vi "TCPIPmain.vi"(5 "data":T1, 6 "config":T3, 7 "error in":errorcluster, 8 "data in":string, 9 "targer":enum16{"driver", "loader"}(ring), 10 "Enum":T4) -> (0 "error out":errorcluster, 1 "LED":bool[](array[boolean]), 2 "data out":T1, 3 "Data?":bool[](array[boolean]))   [LabVIEW 2015]
uses:
  TCPIP_enum.ctl
  TCPIPconfig.ctl
  Ctrls/data out array.ctl
  Ctrls/data out.ctl
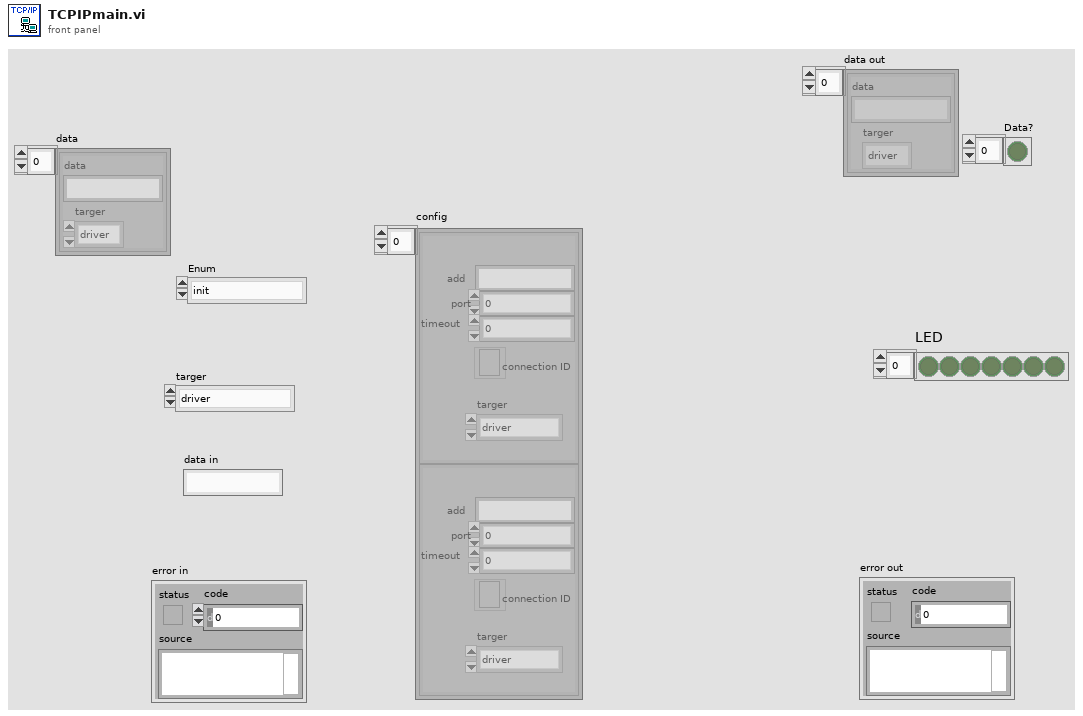
[diagram p1: front panel]
types:
  T1 = typedef "data out array.ctl" = T2[]
  T2 = typedef "data out.ctl" = cluster{"data":string, "targer":enum16{"driver", "loader"}}
  T3 = typedef "TCPIPconfig.ctl" = cluster{"add":string, "port":u32, "timeout":u16, "connection ID":refnum<k5>, "targer":enum16{"driver", "loader"}}[]
  T4 = typedef "TCPIP_enum.ctl" = enum16{"init", "connect", "command", "write", "read", "close", "null"}
  T5 = cluster{"data":string, "targer":enum16{"driver", "loader"}}
  T6 = cluster{"add":string, "port":u32, "timeout":u16, "connection ID":refnum<k5>, "targer":enum16{"driver", "loader"}}
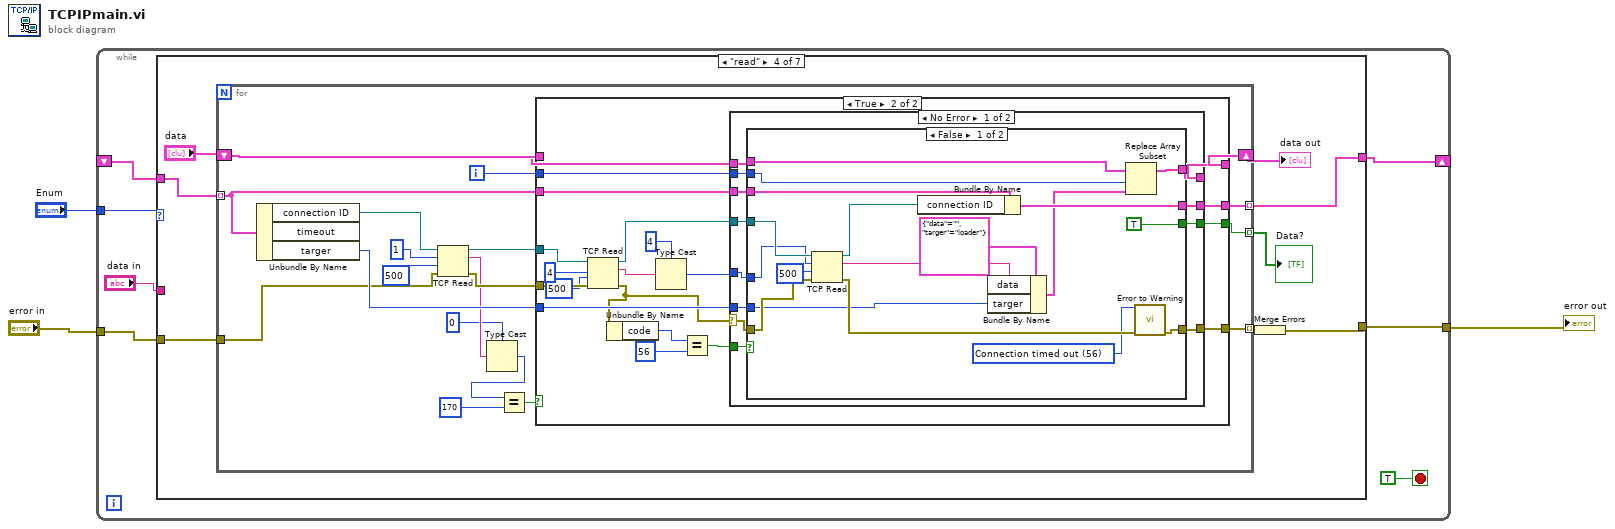
[diagram p0: block diagram]
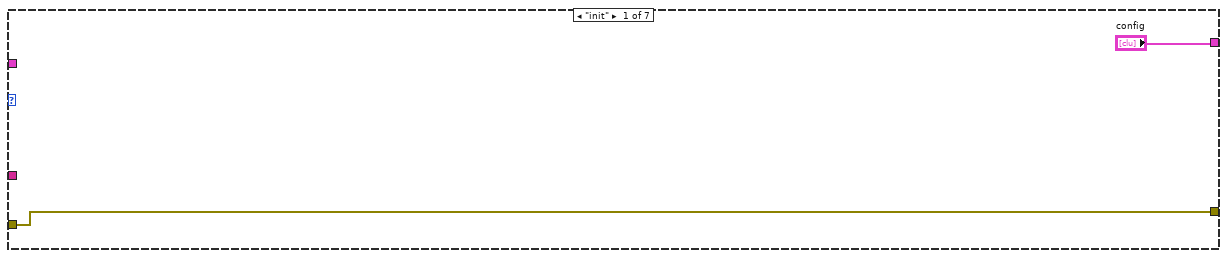
[diagram p2: hidden frame]
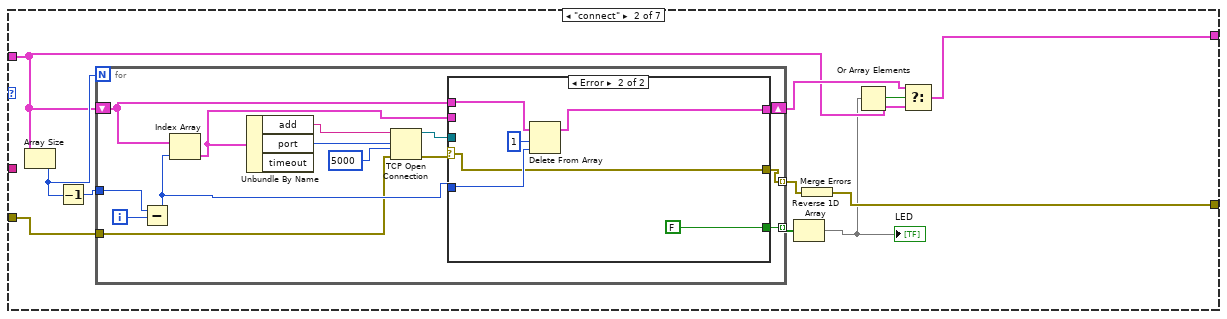
[diagram p3: hidden frame]
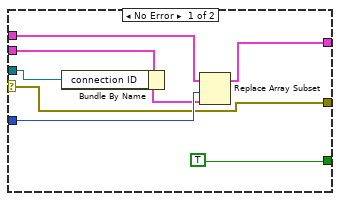
[diagram p4: hidden frame]
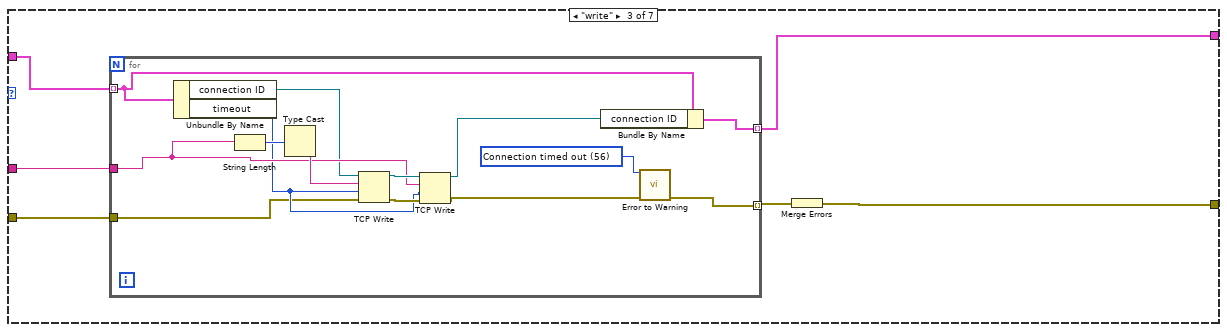
[diagram p5: hidden frame]
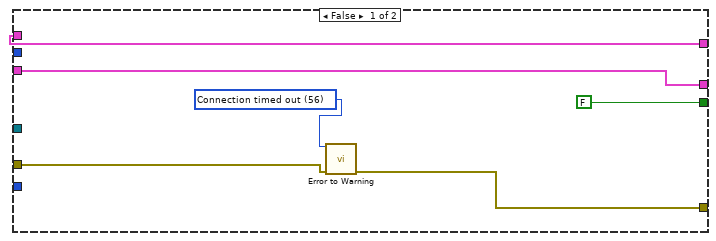
[diagram p6: hidden frame]
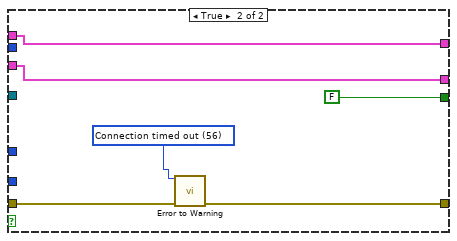
[diagram p7: hidden frame]
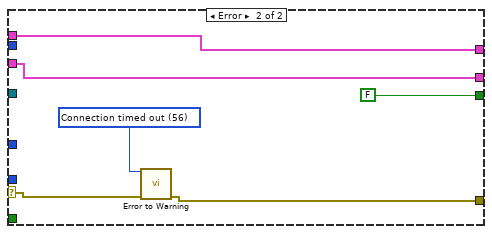
[diagram p8: hidden frame]
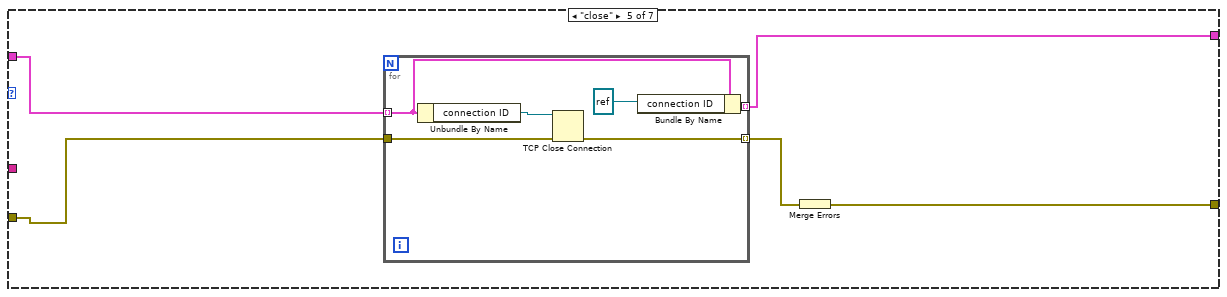
[diagram p9: hidden frame]
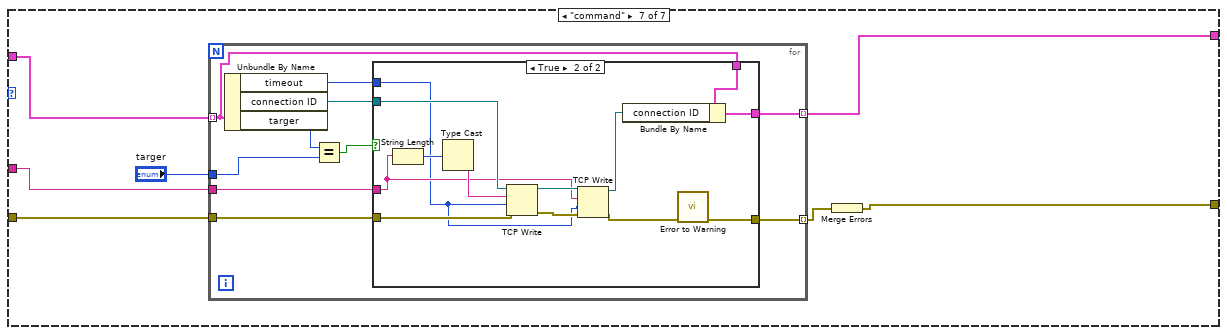
[diagram p11: hidden frame]
diagram:
  n1 = while {
    shift-right: [w8] -> _
    shift-left: _ -> [w7]
    tunnel: [w6] -> w2
    tunnel: "error in" -> [w5]
    tunnel: "Enum" -> [w9]
    stop <- TRUE stop-if-true
    n2 = case shown="\"read\"" w9 {
      tunnel: ["config" w14 w56 w78 w167 w179 w182] -> w8
      tunnel: w7 -> [_ w15 w57 w79 w171 w179 w186]
      tunnel: [w11 w20 w54 w76 w168 w178 w181] -> w6
      tunnel: w5 -> [w11 w22 w53 w75 w170 w178 w184]
      tunnel: "data in" -> [_ _ w52 _ _ _ w183]
      frame "init" {
      }
      frame "connect" {
        n3 = Array Size(array=w15) -> (size(s)=w19:i32)
        n4 = Decrement(x=w19) -> (x-1=w23:i32)
        n5 = for {
          N: w19 -> [_]
          shift-right: [w29] -> w16
          shift-left: w15 -> [w33]
          tunnel: w23 -> [w31]
          tunnel: w22 -> [w28]
          tunnel: [w27] -> w21 mode=indexing
          tunnel: [w26] -> w18 mode=indexing
          i -> [w32]
          n6 = Subtract(x=w31, y=w32) -> (x-y=w30:i32)
          n7 = Index Array(array=w33, index=w30) -> (element=w34:T6)
          n8 = Unbundle By Name(w34) -> ("add"=w37:string, "port"=w25:u32)  [unwired: 1 out]
          n9 = TCP Open Connection(address=w37, remote port or service name=w25, timeout ms (60000)=5000, error in (no error)=w28) -> (connection ID=w36:refnum<k5>, error out=w35:errorcluster)  [unwired: 1 in]
          n10 = case shown="Error" w35 {
            selector: w35 -> [w39 w47]
            tunnel: w36 -> [w45 _]
            tunnel: w34 -> [w44 _]
            tunnel: w33 -> [w43 w51]
            tunnel: w30 -> [w42 w49]
            tunnel: [w40 w48] -> w29
            tunnel: [w39 w47] -> w27
            tunnel: [TRUE FALSE] -> w26
            frame No Error {
              n11 = Bundle By Name(cluster=w44, "connection ID"=w45) -> (w41:T6)
              n12 = Replace Array Subset "Replace Array Subset"(array=w43, new element=w41, index=w42) -> (w40:T3)
            }
            frame Error {
              n13 = Delete From Array(array=w51, length=1, index=w49) -> (array with subset deleted=w48:T3)  [unwired: 1 out]
            }
          }
        }
        n14 = Reverse 1D Array(array=w18) -> (reversed array=w13:bool[])
        "LED" <- w13
        n15 = Merge Errors(w21) -> (w20:errorcluster)
        n16 = Or Array Elements(Boolean array=w13) -> (logical OR=w17:bool)
        n17 = Select(t=w16, s=w17, f=w15) -> (s? t:f=w14:T3)
      }
      frame "write" {
        n18 = for {
          tunnel: w57 -> [w63] mode=indexing
          tunnel: w52 -> [w66]
          tunnel: [w61] -> w56 mode=indexing
          tunnel: [w60] -> w55 mode=indexing
          tunnel: w53 -> [w59]
          w58 = 56 items=["No Error", "Argument Error", "Memory Full", "Out of Zone", "End of File", "File Already Open", "Generic File IO Error", "File Not Found", "File Permission Error", "Disk Full", "Duplicate Path", "Too Many Files Open", "Not Enabled", "Resource File Not Found", "Cannot Add Resource", "Resource Not Found", "Image Not Found", "Image Memory Error", "Pen Does Not Exist", "Config Bad Type", "Config Token Not Found", "Config Parse Error", "Config Memory Error", "Bad External Code Format", "Bad External Code Offset", "External Code Not Present", "Null Window", "Destroy Window Mixup", "Null Menu", "Print Aborted", "Bad Print Record", "Print Driver Error", "Windows Error During Print", "Memory Error During Print", "Print Dialog Error", "Generic Print Error", "Invalid Device Refnum", "Device Not Found", "Device Parameter Error", "Device Unit Error", "Can't Open Device", "Device Call Aborted", "Generic Error", "Cancelled By User", "Object ID Too Low", "Object ID Too High", "Object Not In Heap", "Unknown Heap", "Bad DefProc ID", "DefProc Not In Table", "Message Out Of Range", "Null Method", "Unknown Message", "Manager Call Not Supported", "Bad address", "Connection In progress", "Connection timed out", "Connection is already in progress", "Network attribute not supported", "Network error", "Address in use", "System out of memory", "Connection aborted", "Connection refused", "Connection is not connected", "Connection is already connected", "Connection closed", "Initialize error (interapplication manager)", "Bad occurrence", "Wait on unbound occurrence handler", "Occurrence queue overflow", "Bad path", "Semaphore not signaled", "Unrecognized type (interapplication manager)"] ("1st Error to Convert")
          n19 = Unbundle By Name(w63) -> ("connection ID"=w65:refnum<k5>, "timeout"=w64:u16)
          n20 = String Length(string=w66) -> (length=w71:i32)
          n21 = Type Cast(x=w71) -> (*(type *) &x=w68:string)  [unwired: 1 out]
          n22 = TCP Write(connection ID=w65, data in=w68, error in (no error)=w59, 9:w64) -> (connection ID out=w70:refnum<k5>, error out=w69:errorcluster)  [unwired: 1 out]
          n23 = TCP Write(connection ID=w70, data in=w66, error in (no error)=w69, 9:w64) -> (connection ID out=w62:refnum<k5>, error out=w67:errorcluster)  [unwired: 1 out]
          n24 = Bundle By Name(cluster=w63, "connection ID"=w62) -> (w61:T6)
          n25 = call <vilib>:"Error to Warning.vi"("1st Error to Convert"=w58, "error in"=w67) -> ("warning out"=w60:errorcluster)  [unwired: 4 in, 9 out]
        }
        n26 = Merge Errors(w55) -> (w54:errorcluster)
      }
      frame "read" {
        n27 = for {
          tunnel: w79 -> [w98] mode=indexing
          tunnel: [w97] -> w78 mode=indexing
          tunnel: [w96] -> w77 mode=indexing
          tunnel: w75 -> [w94]
          shift-right: [w83] -> w72
          shift-left: "data" -> [w84]
          tunnel: [w81] -> w73 mode=indexing
          i -> [w82]
          n28 = Unbundle By Name(w98) -> ("connection ID"=w93:refnum<k5>, "targer"=w95:enum16{"driver", "loader"})  [unwired: 1 out]
          n29 = TCP Read(connection ID=w93, bytes to read=1, error in (no error)=w94, 9:500 ("timeout ms (25000)")) -> (connection ID out=w90:refnum<k5>, data out=w89:string, error out=w91:errorcluster)  [unwired: 1 out]
          n30 = Type Cast(type=u8 0, x=w89) -> (*(type *) &x=w87:u8)
          n31 = Equal?(x=w87, y=u8 170) -> (x = y?=w85:bool)
          n32 = case shown="True" w85 {
            tunnel: w90 -> [_ w120]
            tunnel: w98 -> [w104 w119]
            tunnel: [w104 w118] -> w97
            tunnel: [w100 w117] -> w96
            tunnel: w91 -> [w101 w116]
            tunnel: w95 -> [_ w115]
            tunnel: w84 -> [w103 w109]
            tunnel: [w103 w108] -> w83
            tunnel: w82 -> [_ w107]
            tunnel: [FALSE w106] -> w81
            frame False {
              w99 = 56 items=["No Error", "Argument Error", "Memory Full", "Out of Zone", "End of File", "File Already Open", "Generic File IO Error", "File Not Found", "File Permission Error", "Disk Full", "Duplicate Path", "Too Many Files Open", "Not Enabled", "Resource File Not Found", "Cannot Add Resource", "Resource Not Found", "Image Not Found", "Image Memory Error", "Pen Does Not Exist", "Config Bad Type", "Config Token Not Found", "Config Parse Error", "Config Memory Error", "Bad External Code Format", "Bad External Code Offset", "External Code Not Present", "Null Window", "Destroy Window Mixup", "Null Menu", "Print Aborted", "Bad Print Record", "Print Driver Error", "Windows Error During Print", "Memory Error During Print", "Print Dialog Error", "Generic Print Error", "Invalid Device Refnum", "Device Not Found", "Device Parameter Error", "Device Unit Error", "Can't Open Device", "Device Call Aborted", "Generic Error", "Cancelled By User", "Object ID Too Low", "Object ID Too High", "Object Not In Heap", "Unknown Heap", "Bad DefProc ID", "DefProc Not In Table", "Message Out Of Range", "Null Method", "Unknown Message", "Manager Call Not Supported", "Bad address", "Connection In progress", "Connection timed out", "Connection is already in progress", "Network attribute not supported", "Network error", "Address in use", "System out of memory", "Connection aborted", "Connection refused", "Connection is not connected", "Connection is already connected", "Connection closed", "Initialize error (interapplication manager)", "Bad occurrence", "Wait on unbound occurrence handler", "Occurrence queue overflow", "Bad path", "Semaphore not signaled", "Unrecognized type (interapplication manager)"] ("1st Error to Convert")
              n33 = call <vilib>:"Error to Warning.vi"("1st Error to Convert"=w99, "error in"=w101) -> ("warning out"=w100:errorcluster)  [unwired: 4 in, 9 out]
            }
            frame True {
              n34 = TCP Read(connection ID=w120, bytes to read=4, error in (no error)=w116, 9:500 ("timeout ms (25000)")) -> (connection ID out=w123:refnum<k5>, data out=w124:string, error out=w110:errorcluster)  [unwired: 1 out]
              n35 = Unbundle By Name(w110) -> ("code"=w113:i32)
              n36 = Type Cast(type=4, x=w124) -> (*(type *) &x=w122:i32)
              n37 = Equal?(x=w113, y=56) -> (x = y?=w111:bool)
              n38 = case shown="No Error" w110 {
                selector: w110 -> [w125 w163]
                tunnel: w123 -> [w136 _]
                tunnel: w122 -> [w135 _]
                tunnel: w119 -> [w134 w166]
                tunnel: [w133 w166] -> w118
                tunnel: [w132 w162] -> w117
                tunnel: w115 -> [w131 _]
                tunnel: w111 -> [w130 _]
                tunnel: w109 -> [w129 w165]
                tunnel: [w128 w165] -> w108
                tunnel: w107 -> [w127 _]
                tunnel: [w126 FALSE] -> w106
                frame No Error {
                  n39 = case shown="False" w130 {
                    tunnel: w136 -> [w154 _]
                    tunnel: w135 -> [w153 _]
                    tunnel: w134 -> [w150 w160]
                    tunnel: [w149 w160] -> w133
                    tunnel: [w147 w157] -> w132
                    tunnel: w131 -> [w138 _]
                    tunnel: w129 -> [w144 w159]
                    tunnel: [w143 w159] -> w128
                    tunnel: w127 -> [w141 _]
                    tunnel: [TRUE FALSE] -> w126
                    tunnel: w125 -> [w139 w155]
                    frame False {
                      w151 = 56 items=["No Error", "Argument Error", "Memory Full", "Out of Zone", "End of File", "File Already Open", "Generic File IO Error", "File Not Found", "File Permission Error", "Disk Full", "Duplicate Path", "Too Many Files Open", "Not Enabled", "Resource File Not Found", "Cannot Add Resource", "Resource Not Found", "Image Not Found", "Image Memory Error", "Pen Does Not Exist", "Config Bad Type", "Config Token Not Found", "Config Parse Error", "Config Memory Error", "Bad External Code Format", "Bad External Code Offset", "External Code Not Present", "Null Window", "Destroy Window Mixup", "Null Menu", "Print Aborted", "Bad Print Record", "Print Driver Error", "Windows Error During Print", "Memory Error During Print", "Print Dialog Error", "Generic Print Error", "Invalid Device Refnum", "Device Not Found", "Device Parameter Error", "Device Unit Error", "Can't Open Device", "Device Call Aborted", "Generic Error", "Cancelled By User", "Object ID Too Low", "Object ID Too High", "Object Not In Heap", "Unknown Heap", "Bad DefProc ID", "DefProc Not In Table", "Message Out Of Range", "Null Method", "Unknown Message", "Manager Call Not Supported", "Bad address", "Connection In progress", "Connection timed out", "Connection is already in progress", "Network attribute not supported", "Network error", "Address in use", "System out of memory", "Connection aborted", "Connection refused", "Connection is not connected", "Connection is already connected", "Connection closed", "Initialize error (interapplication manager)", "Bad occurrence", "Wait on unbound occurrence handler", "Occurrence queue overflow", "Bad path", "Semaphore not signaled", "Unrecognized type (interapplication manager)"] ("1st Error to Convert")
                      n40 = TCP Read(connection ID=w154, bytes to read=w153, error in (no error)=w139, 9:500 ("timeout ms (25000)")) -> (connection ID out=w148:refnum<k5>, data out=w145:string, error out=w152:errorcluster)  [unwired: 1 out]
                      n41 = Bundle By Name(cluster=w150, "connection ID"=w148) -> (w149:T6)
                      n42 = Bundle By Name(cluster=T5 {"data"="", "targer"=enum."loader"} ("data out"), "data"=w145, "targer"=w138) -> (w142:T5)
                      n43 = Replace Array Subset(array=w144, new element=w142, index=w141) -> (w143:T1)
                      n44 = call <vilib>:"Error to Warning.vi"("1st Error to Convert"=w151, "error in"=w152) -> ("warning out"=w147:errorcluster)  [unwired: 4 in, 9 out]
                    }
                    frame True {
                      w156 = 56 items=["No Error", "Argument Error", "Memory Full", "Out of Zone", "End of File", "File Already Open", "Generic File IO Error", "File Not Found", "File Permission Error", "Disk Full", "Duplicate Path", "Too Many Files Open", "Not Enabled", "Resource File Not Found", "Cannot Add Resource", "Resource Not Found", "Image Not Found", "Image Memory Error", "Pen Does Not Exist", "Config Bad Type", "Config Token Not Found", "Config Parse Error", "Config Memory Error", "Bad External Code Format", "Bad External Code Offset", "External Code Not Present", "Null Window", "Destroy Window Mixup", "Null Menu", "Print Aborted", "Bad Print Record", "Print Driver Error", "Windows Error During Print", "Memory Error During Print", "Print Dialog Error", "Generic Print Error", "Invalid Device Refnum", "Device Not Found", "Device Parameter Error", "Device Unit Error", "Can't Open Device", "Device Call Aborted", "Generic Error", "Cancelled By User", "Object ID Too Low", "Object ID Too High", "Object Not In Heap", "Unknown Heap", "Bad DefProc ID", "DefProc Not In Table", "Message Out Of Range", "Null Method", "Unknown Message", "Manager Call Not Supported", "Bad address", "Connection In progress", "Connection timed out", "Connection is already in progress", "Network attribute not supported", "Network error", "Address in use", "System out of memory", "Connection aborted", "Connection refused", "Connection is not connected", "Connection is already connected", "Connection closed", "Initialize error (interapplication manager)", "Bad occurrence", "Wait on unbound occurrence handler", "Occurrence queue overflow", "Bad path", "Semaphore not signaled", "Unrecognized type (interapplication manager)"] ("1st Error to Convert")
                      n45 = call <vilib>:"Error to Warning.vi"("1st Error to Convert"=w156, "error in"=w155) -> ("warning out"=w157:errorcluster)  [unwired: 4 in, 9 out]
                    }
                  }
                }
                frame Error {
                  w161 = 56 items=["No Error", "Argument Error", "Memory Full", "Out of Zone", "End of File", "File Already Open", "Generic File IO Error", "File Not Found", "File Permission Error", "Disk Full", "Duplicate Path", "Too Many Files Open", "Not Enabled", "Resource File Not Found", "Cannot Add Resource", "Resource Not Found", "Image Not Found", "Image Memory Error", "Pen Does Not Exist", "Config Bad Type", "Config Token Not Found", "Config Parse Error", "Config Memory Error", "Bad External Code Format", "Bad External Code Offset", "External Code Not Present", "Null Window", "Destroy Window Mixup", "Null Menu", "Print Aborted", "Bad Print Record", "Print Driver Error", "Windows Error During Print", "Memory Error During Print", "Print Dialog Error", "Generic Print Error", "Invalid Device Refnum", "Device Not Found", "Device Parameter Error", "Device Unit Error", "Can't Open Device", "Device Call Aborted", "Generic Error", "Cancelled By User", "Object ID Too Low", "Object ID Too High", "Object Not In Heap", "Unknown Heap", "Bad DefProc ID", "DefProc Not In Table", "Message Out Of Range", "Null Method", "Unknown Message", "Manager Call Not Supported", "Bad address", "Connection In progress", "Connection timed out", "Connection is already in progress", "Network attribute not supported", "Network error", "Address in use", "System out of memory", "Connection aborted", "Connection refused", "Connection is not connected", "Connection is already connected", "Connection closed", "Initialize error (interapplication manager)", "Bad occurrence", "Wait on unbound occurrence handler", "Occurrence queue overflow", "Bad path", "Semaphore not signaled", "Unrecognized type (interapplication manager)"] ("1st Error to Convert")
                  n46 = call <vilib>:"Error to Warning.vi"("1st Error to Convert"=w161, "error in"=w163) -> ("warning out"=w162:errorcluster)  [unwired: 4 in, 9 out]
                }
              }
            }
          }
        }
        "Data?" <- w73
        "data out" <- w72
        n47 = Merge Errors(w77) -> (w76:errorcluster)
      }
      frame "close" {
        n48 = for {
          tunnel: w171 -> [w174] mode=indexing
          tunnel: w170 -> [w176]
          tunnel: [w175] -> w169 mode=indexing
          tunnel: [w172] -> w167 mode=indexing
          n49 = Unbundle By Name(w174) -> ("connection ID"=w177:refnum<k5>)
          n50 = TCP Close Connection(connection ID=w177, error in (no error)=w176) -> (error out=w175:errorcluster)  [unwired: 2 out]
          n51 = Bundle By Name(cluster=w174, "connection ID"=refnum<k5> refnum) -> (w172:T6)
        }
        n52 = Merge Errors(w169) -> (w168:errorcluster)
      }
      frame "null", Default {
      }
      frame "command" {
        n53 = for {
          tunnel: w186 -> [w188] mode=indexing
          tunnel: "targer" -> [w195]
          tunnel: w184 -> [w192]
          tunnel: [w191] -> w180 mode=indexing
          tunnel: w183 -> [w190]
          tunnel: [w187] -> w182 mode=indexing
          n54 = Unbundle By Name(w188) -> ("timeout"=w189:u16, "connection ID"=w193:refnum<k5>, "targer"=w196:enum16{"driver", "loader"})
          n55 = Equal?(x=w196, y=w195) -> (x = y?=w194:bool)
          n56 = case shown="True" w194 {
            tunnel: w193 -> [_ w206]
            tunnel: w192 -> [w197 w205]
            tunnel: [w197 w204] -> w191
            tunnel: w190 -> [_ w203]
            tunnel: w189 -> [_ w202]
            tunnel: w188 -> [w198 w201]
            tunnel: [w198 w199] -> w187
            frame False {
            }
            frame True {
              n57 = String Length(string=w203) -> (length=w211:i32)
              n58 = Type Cast(x=w211) -> (*(type *) &x=w208:string)  [unwired: 1 out]
              n59 = TCP Write(connection ID=w206, data in=w208, error in (no error)=w205, 9:w202) -> (connection ID out=w210:refnum<k5>, error out=w209:errorcluster)  [unwired: 1 out]
              n60 = TCP Write(connection ID=w210, data in=w203, error in (no error)=w209, 9:w202) -> (connection ID out=w200:refnum<k5>, error out=w207:errorcluster)  [unwired: 1 out]
              n61 = Bundle By Name(cluster=w201, "connection ID"=w200) -> (w199:T6)
              n62 = call <vilib>:"Error to Warning.vi"("error in"=w207) -> ("warning out"=w204:errorcluster)  [unwired: 5 in, 9 out]
            }
          }
        }
        n63 = Merge Errors(w180) -> (w181:errorcluster)
      }
    }
  }
  "error out" <- w2
